vi "HFRR ADV v024 new software.vi"() -> ()   [LabVIEW 2025] (continued)
              n2182 = Fract/Exp String To Number(string=w2595) -> (number=w2598:dbl)  [unwired: 3 in, 1 out]
              n2183 = Add(x=w2598, y=0.0) -> (x+y=w2594:dbl)
            }
            n2184 = for {
              N: w2486 -> [_]
              tunnel: w2493 -> [w2541]
              tunnel: w2492 -> [w2540]
              tunnel: [w2530] -> w2446 mode=indexing
              tunnel: [w2529] -> w2439 mode=indexing
              tunnel: w2483 -> [_]
              tunnel: [w2518] -> w2444 mode=indexing
              tunnel: [w2523] -> w2441 mode=indexing
              tunnel: [w2519] -> w2431 mode=indexing
              tunnel: [w2514] -> w2406 mode=indexing
              tunnel: [w2510] -> w2387 mode=indexing
              tunnel: [w2505] -> w2347 mode=indexing
              (unwired) 1.0 ("x")
              (unwired) TRUE ("line mode (F)")
              n2185 = Read from Text File "Read File"(file (use dialog)=w2541, error in=w2540) -> (text=w2506:string)  [unwired: 2 in, 3 out]
              n2186 = local write "String 12"(w2506) -> ()
              n2187 = String Subset(string=w2506, offset (0)=85, length (rest)=9 ("length (rest)")) -> (substring=w2508:string)
              n2188 = String Subset(string=w2506, offset (0)=35, length (rest)=9 ("length (rest)")) -> (substring=w2531:string)
              n2189 = String Subset(string=w2506, offset (0)=55, length (rest)=9 ("length (rest)")) -> (substring=w2516:string)
              n2190 = String Subset(string=w2506, offset (0)=25, length (rest)=9 ("length (rest)")) -> (substring=w2512:string)
              n2191 = String Subset(string=w2506, offset (0)=45, length (rest)=9 ("length (rest)")) -> (substring=w2521:string)
              n2192 = String Subset(string=w2506, offset (0)=15, length (rest)=9 ("length (rest)")) -> (substring=w2537:string)
              n2193 = String Subset(string=w2506, offset (0)=0, length (rest)=14 ("length (rest)")) -> (substring=w2534:string)
              n2194 = String Subset(string=w2506, offset (0)=65, length (rest)=9 ("length (rest)")) -> (substring=w2524:string)
              n2195 = Fract/Exp String To Number(string=w2508) -> (number=w2505:dbl)  [unwired: 3 in, 1 out]
              n2196 = Fract/Exp String To Number(string=w2531) -> (number=w2529:dbl)  [unwired: 3 in, 1 out]
              n2197 = Fract/Exp String To Number(string=w2516) -> (number=w2514:dbl)  [unwired: 3 in, 1 out]
              n2198 = Fract/Exp String To Number(string=w2512) -> (number=w2510:dbl)  [unwired: 3 in, 1 out]
              n2199 = Fract/Exp String To Number(string=w2521) -> (number=w2519:dbl)  [unwired: 3 in, 1 out]
              n2200 = Fract/Exp String To Number(string=w2537) -> (number=w2518:dbl)  [unwired: 3 in, 1 out]
              n2201 = Fract/Exp String To Number(string=w2534) -> (number=w2530:dbl)  [unwired: 3 in, 1 out]
              n2202 = Fract/Exp String To Number(string=w2524) -> (number=w2527:dbl)  [unwired: 3 in, 1 out]
              n2203 = Add(x=w2527, y=0.0) -> (x+y=w2523:dbl)
            }
            n2204 = Delete From Array(array=w2389, index=0) -> (array with subset deleted=w2362:dbl[])  [unwired: 1 in, 1 out]
            n2205 = Delete From Array(array=w2452, index=0) -> (array with subset deleted=w2425:dbl[])  [unwired: 1 in, 1 out]
            n2206 = Delete From Array(array=w2432, index=0) -> (array with subset deleted=w2420:dbl[])  [unwired: 1 in, 1 out]
            n2207 = Delete From Array(array=w2450, index=0) -> (array with subset deleted=w2451:dbl[])  [unwired: 1 in, 1 out]
            n2208 = call-poly <vilib>:"Mean.vi"("X"=w2362) -> ("mean"=→"КОФ2 4":dbl)  [unwired: 1 out]
            n2209 = call-poly <vilib>:"Mean.vi"("X"=w2425) -> ("mean"=→"КОФ3":dbl)  [unwired: 1 out]
            n2210 = call-poly <vilib>:"Mean.vi"("X"=w2420) -> ("mean"=→"CP3":dbl)  [unwired: 1 out]
            n2211 = Delete From Array(array=w2414, index=0) -> (array with subset deleted=w2341:dbl[])  [unwired: 1 in, 1 out]
            n2212 = Delete From Array(array=w2353, index=0) -> (array with subset deleted=w2340:dbl[])  [unwired: 1 in, 1 out]
            n2213 = Delete From Array(array=w2393, index=0) -> (array with subset deleted=w2364:dbl[])  [unwired: 1 in, 1 out]
            n2214 = Delete From Array(array=w2471, index=0) -> (array with subset deleted=w2426:dbl[])  [unwired: 1 in, 1 out]
            n2215 = Delete From Array(array=w2437, index=0) -> (array with subset deleted=w2422:dbl[])  [unwired: 1 in, 1 out]
            "array w/ subset deleted" <- w2422
            n2216 = Delete From Array(array=w2468, index=0) -> (array with subset deleted=w2469:dbl[])  [unwired: 1 in, 1 out]
            n2217 = call-poly <vilib>:"Mean.vi"("X"=w2364) -> ("mean"=→"КОФ2 2":dbl)  [unwired: 1 out]
            n2218 = call-poly <vilib>:"Mean.vi"("X"=w2426) -> ("mean"=→"КОФ1":dbl)  [unwired: 1 out]
            n2219 = Bundle "Bundle"(w2341, w2340) -> (w2346:cluster{dbl[], dbl[]})  [unwired: 1 in]
            n2220 = Bundle "Bundle"(w2341, w2469) -> (w2333:cluster{dbl[], dbl[]})  [unwired: 1 in]
            n2221 = Delete From Array(array=w2348, index=0) -> (array with subset deleted=w2336:dbl[])  [unwired: 1 in, 1 out]
            n2222 = Delete From Array(array=w2349, index=0) -> (array with subset deleted=w2338:dbl[])  [unwired: 1 in, 1 out]
            n2223 = Delete From Array(array=w2459, index=0) -> (array with subset deleted=w2460:dbl[])  [unwired: 1 in, 1 out]
            n2224 = Delete From Array(array=w2347, index=0) -> (array with subset deleted=w2334:dbl[])  [unwired: 1 in, 1 out]
            n2225 = Delete From Array(array=w2441, index=0) -> (array with subset deleted=w2442:dbl[])  [unwired: 1 in, 1 out]
            n2226 = Delete From Array(array=w2466, index=0) -> (array with subset deleted=w2372:dbl[])  [unwired: 1 in, 1 out]
            n2227 = Delete From Array(array=w2412, index=0) -> (array with subset deleted=w2368:dbl[])  [unwired: 1 in, 1 out]
            n2228 = Delete From Array(array=w2448, index=0) -> (array with subset deleted=w2370:dbl[])  [unwired: 1 in, 1 out]
            n2229 = Delete From Array(array=w2408, index=0) -> (array with subset deleted=w2366:dbl[])  [unwired: 1 in, 1 out]
            n2230 = Delete From Array(array=w2457, index=0) -> (array with subset deleted=w2371:dbl[])  [unwired: 1 in, 1 out]
            n2231 = Delete From Array(array=w2410, index=0) -> (array with subset deleted=w2367:dbl[])  [unwired: 1 in, 1 out]
            n2232 = Delete From Array(array=w2391, index=0) -> (array with subset deleted=w2363:dbl[])  [unwired: 1 in, 1 out]
            n2233 = Delete From Array(array=w2435, index=0) -> (array with subset deleted=w2421:dbl[])  [unwired: 1 in, 1 out]
            n2234 = Delete From Array(array=w2462, index=0) -> (array with subset deleted=w2423:dbl[])  [unwired: 1 in, 1 out]
            n2235 = Delete From Array(array=w2439, index=0) -> (array with subset deleted=w2369:dbl[])  [unwired: 1 in, 1 out]
            n2236 = Delete From Array(array=w2406, index=0) -> (array with subset deleted=w2365:dbl[])  [unwired: 1 in, 1 out]
            n2237 = Delete From Array(array=w2387, index=0) -> (array with subset deleted=w2361:dbl[])  [unwired: 1 in, 1 out]
            n2238 = Delete From Array(array=w2431, index=0) -> (array with subset deleted=w2419:dbl[])  [unwired: 1 in, 1 out]
            n2239 = Delete From Array(array=w2444, index=0) -> (array with subset deleted=w2424:dbl[])  [unwired: 1 in, 1 out]
            n2240 = Delete From Array(array=w2454, index=0) -> (array with subset deleted=w2337:dbl[])  [unwired: 1 in, 1 out]
            n2241 = Delete From Array(array=w2464, index=0) -> (array with subset deleted=w2339:dbl[])  [unwired: 1 in, 1 out]
            n2242 = Delete From Array(array=w2446, index=0) -> (array with subset deleted=w2335:dbl[])  [unwired: 1 in, 1 out]
            n2243 = Bundle "Bundle"(w2341, w2372) -> (w2359:cluster{dbl[], dbl[]})  [unwired: 1 in]
            n2244 = Bundle "Bundle"(w2341, w2426) -> (w2360:cluster{dbl[], dbl[]})  [unwired: 1 in]
            n2245 = Bundle "Bundle"(w2372, w2368) -> (w2374:cluster{dbl[], dbl[]})  [unwired: 1 in]
            n2246 = Bundle "Bundle"(w2337, w2336) -> (w2344:cluster{dbl[], dbl[]})  [unwired: 1 in]
            n2247 = Bundle "Bundle"(w2370, w2366) -> (w2376:cluster{dbl[], dbl[]})  [unwired: 1 in]
            n2248 = Bundle "Bundle"(w2337, w2370) -> (w2480:cluster{dbl[], dbl[]})  [unwired: 1 in]
            n2249 = Bundle "Bundle"(w2337, w2366) -> (w2404:cluster{dbl[], dbl[]})  [unwired: 1 in]
            n2250 = Bundle "Bundle"(w2337, w2425) -> (w2490:cluster{dbl[], dbl[]})  [unwired: 1 in]
            n2251 = Bundle "Bundle"(w2337, w2420) -> (w2428:cluster{dbl[], dbl[]})  [unwired: 1 in]
            n2252 = Bundle "Bundle"(w2337, w2451) -> (w2475:cluster{dbl[], dbl[]})  [unwired: 1 in]
            n2253 = Bundle "Bundle"(w2371, w2367) -> (w2375:cluster{dbl[], dbl[]})  [unwired: 1 in]
            n2254 = Bundle "Bundle"(w2339, w2338) -> (w2345:cluster{dbl[], dbl[]})  [unwired: 1 in]
            n2255 = Bundle "Bundle"(w2339, w2371) -> (w2482:cluster{dbl[], dbl[]})  [unwired: 1 in]
            n2256 = Bundle "Bundle"(w2339, w2367) -> (w2405:cluster{dbl[], dbl[]})  [unwired: 1 in]
            n2257 = Bundle "Bundle"(w2339, w2421) -> (w2429:cluster{dbl[], dbl[]})  [unwired: 1 in]
            n2258 = Bundle "Bundle"(w2339, w2423) -> (w2491:cluster{dbl[], dbl[]})  [unwired: 1 in]
            n2259 = Bundle "Bundle"(w2339, w2460) -> (w2473:cluster{dbl[], dbl[]})  [unwired: 1 in]
            n2260 = Bundle "Bundle"(w2369, w2365) -> (w2377:cluster{dbl[], dbl[]})  [unwired: 1 in]
            n2261 = Bundle "Bundle"(w2335, w2334) -> (w2343:cluster{dbl[], dbl[]})  [unwired: 1 in]
            n2262 = Bundle "Bundle"(w2335, w2369) -> (w2481:cluster{dbl[], dbl[]})  [unwired: 1 in]
            n2263 = Bundle "Bundle"(w2335, w2365) -> (w2403:cluster{dbl[], dbl[]})  [unwired: 1 in]
            n2264 = Bundle "Bundle"(w2335, w2419) -> (w2427:cluster{dbl[], dbl[]})  [unwired: 1 in]
            n2265 = Bundle "Bundle"(w2335, w2424) -> (w2489:cluster{dbl[], dbl[]})  [unwired: 1 in]
            n2266 = Bundle "Bundle"(w2335, w2442) -> (w2474:cluster{dbl[], dbl[]})  [unwired: 1 in]
            n2267 = call-poly <vilib>:"Mean.vi"("X"=w2422) -> ("mean"=→"CP1":dbl)  [unwired: 1 out]
            n2268 = call-poly <vilib>:"Mean.vi"("X"=w2363) -> ("mean"=→"КОФ2 3":dbl)  [unwired: 1 out]
            n2269 = call-poly <vilib>:"Mean.vi"("X"=w2421) -> ("mean"=→"CP2":dbl)  [unwired: 1 out]
            n2270 = call-poly <vilib>:"Mean.vi"("X"=w2423) -> ("mean"=→"КОФ2":dbl)  [unwired: 1 out]
            n2271 = call-poly <vilib>:"Mean.vi"("X"=w2361) -> ("mean"=→"КОФ2 5":dbl)  [unwired: 1 out]
            n2272 = call-poly <vilib>:"Mean.vi"("X"=w2419) -> ("mean"=→"CP4":dbl)  [unwired: 1 out]
            n2273 = call-poly <vilib>:"Mean.vi"("X"=w2424) -> ("mean"=→"КОФ4":dbl)  [unwired: 1 out]
            n2274 = Bundle "Bundle"(w2341, w2368) -> (w2332:cluster{dbl[], dbl[]})  [unwired: 1 in]
            n2275 = Bundle "Bundle"(w2341, w2422) -> (w2355:cluster{dbl[], dbl[]})  [unwired: 1 in]
            n2276 = Build Array "Build Array"(w2332, w2355) -> (w2358:cluster{dbl[], dbl[]}[])
            "XY Graph 17" <- w2358
            n2277 = Build Array "Build Array"(w2346, w2345, w2344, w2343) -> (→"Frequency ( Hz )":cluster{dbl[], dbl[]}[])
            n2278 = Build Array "Build Array"(w2374, w2375, w2376, w2377) -> (→"Air Temp ( °C ) vs Humidity ( % RH )":cluster{dbl[], dbl[]}[])
            n2279 = Build Array "Build Array"(w2359, w2482, w2480, w2481) -> (→"Air Temperature  ( °C )":cluster{dbl[], dbl[]}[])
            n2280 = Build Array "Build Array"(w2332, w2405, w2404, w2403) -> (→"Humidity ( %RH )":cluster{dbl[], dbl[]}[])
            n2281 = Build Array "Build Array"(w2360, w2491, w2490, w2489) -> (→"Coefficient Of Friction":cluster{dbl[], dbl[]}[])
            n2282 = Build Array "Build Array"(w2355, w2429, w2428, w2427) -> (→"Sample Temperature ( °C )":cluster{dbl[], dbl[]}[])
            n2283 = Build Array "Build Array"(w2333, w2473, w2475, w2474) -> (→"XY Graph 13":cluster{dbl[], dbl[]}[])
            n2284 = Bundle "Bundle"(w2341, w2364) -> (w2386:cluster{dbl[], dbl[]})  [unwired: 1 in]
            n2285 = Bundle "Bundle"(w2337, w2362) -> (w2384:cluster{dbl[], dbl[]})  [unwired: 1 in]
            n2286 = Bundle "Bundle"(w2339, w2363) -> (w2385:cluster{dbl[], dbl[]})  [unwired: 1 in]
            n2287 = Bundle "Bundle"(w2335, w2361) -> (w2383:cluster{dbl[], dbl[]})  [unwired: 1 in]
            n2288 = Build Array "Build Array"(w2386, w2385, w2384, w2383) -> (→"Stroke ( mm )":cluster{dbl[], dbl[]}[])
            n2289 = local write "XY Graph 16"(w2358) -> ()
          }
          frame #2 {
          }
          frame #3 {
            n2290 = local write "Numeric 8"(0 ("Numeric 8")) -> ()
            n2291 = local write "Numeric 11"(0 ("Numeric 11")) -> ()
            n2292 = local write "Numeric 12"(0 ("Numeric 12")) -> ()
            n2293 = local write "Numeric 13"(0 ("Numeric 13")) -> ()
            n2294 = property on="OPEN" class="Bool (strict)"("Visible"=TRUE) -> ()  [unwired: 2 in, 2 out]
            n2295 = local read "String Control 2"() -> (w2658:string)
            n2296 = local read "String Control 4"() -> (w2657:string)
            n2297 = local read "String Control 6"() -> (w2656:string)
            n2298 = local read "String Control 8"() -> (w2655:string)
            n2299 = Match Pattern(string=w2658, regular expression="Samples / cycle :- ") -> (after substring=w2672:string)  [unwired: 1 in, 3 out]
            n2300 = Match Pattern(string=w2658, regular expression="Frequency :- ") -> (after substring=w2691:string)  [unwired: 1 in, 3 out]
            n2301 = Match Pattern(string=w2657, regular expression="Samples / cycle :- ") -> (after substring=w2668:string)  [unwired: 1 in, 3 out]
            n2302 = Match Pattern(string=w2657, regular expression="Frequency :- ") -> (after substring=w2686:string)  [unwired: 1 in, 3 out]
            n2303 = Match Pattern(string=w2656, regular expression="Samples / cycle :- ") -> (after substring=w2664:string)  [unwired: 1 in, 3 out]
            n2304 = Match Pattern(string=w2656, regular expression="Frequency :- ") -> (after substring=w2681:string)  [unwired: 1 in, 3 out]
            n2305 = Match Pattern(string=w2655, regular expression="Samples / cycle :- ") -> (after substring=w2660:string)  [unwired: 1 in, 3 out]
            n2306 = Match Pattern(string=w2655, regular expression="Frequency :- ") -> (after substring=w2676:string)  [unwired: 1 in, 3 out]
            n2307 = String Subset(string=w2672, length (rest)=6 ("length (rest)")) -> (substring=w2674:string)  [unwired: 1 in]
            n2308 = String Subset(string=w2691, length (rest)=9 ("length (rest)")) -> (substring=w2693:string)  [unwired: 1 in]
            n2309 = String Subset(string=w2668, length (rest)=6 ("length (rest)")) -> (substring=w2670:string)  [unwired: 1 in]
            n2310 = String Subset(string=w2686, length (rest)=9 ("length (rest)")) -> (substring=w2688:string)  [unwired: 1 in]
            n2311 = String Subset(string=w2664, length (rest)=6 ("length (rest)")) -> (substring=w2666:string)  [unwired: 1 in]
            n2312 = String Subset(string=w2681, length (rest)=9 ("length (rest)")) -> (substring=w2683:string)  [unwired: 1 in]
            n2313 = String Subset(string=w2660, length (rest)=6 ("length (rest)")) -> (substring=w2662:string)  [unwired: 1 in]
            n2314 = String Subset(string=w2676, length (rest)=9 ("length (rest)")) -> (substring=w2678:string)  [unwired: 1 in]
            n2315 = Fract/Exp String To Number(string=w2674) -> (number=w2654:dbl)  [unwired: 3 in, 1 out]
            n2316 = Fract/Exp String To Number(string=w2693) -> (number=w2694:dbl)  [unwired: 3 in, 1 out]
            n2317 = Fract/Exp String To Number(string=w2670) -> (number=w2653:dbl)  [unwired: 3 in, 1 out]
            n2318 = Fract/Exp String To Number(string=w2688) -> (number=w2689:dbl)  [unwired: 3 in, 1 out]
            n2319 = Fract/Exp String To Number(string=w2666) -> (number=w2652:dbl)  [unwired: 3 in, 1 out]
            n2320 = Fract/Exp String To Number(string=w2683) -> (number=w2684:dbl)  [unwired: 3 in, 1 out]
            n2321 = Fract/Exp String To Number(string=w2662) -> (number=w2651:dbl)  [unwired: 3 in, 1 out]
            n2322 = Fract/Exp String To Number(string=w2678) -> (number=w2679:dbl)  [unwired: 3 in, 1 out]
            n2323 = local write "sample1"(w2654) -> ()
            n2324 = local write "freq1"(w2694) -> ()
            n2325 = local write "sample2"(w2653) -> ()
            n2326 = local write "freq2"(w2689) -> ()
            n2327 = local write "sample3"(w2652) -> ()
            n2328 = local write "freq3"(w2684) -> ()
            n2329 = local write "sample4"(w2651) -> ()
            n2330 = local write "freq 4"(w2679) -> ()
          }
        }
      }
    }
    n2331 = case shown="True" w2143 {
      selector: w2143 -> [_ w2271]
      frame False {
      }
      frame True {
        n2332 = Not(x=w2271) -> (.not. x?=w2267:bool)
        n2333 = local write "service 3"(w2267) -> ()
        n2334 = local write "OPEN 6"(w2267) -> ()
        n2335 = call <vilib>:"System Exec.vi"("wait until completion? (T)"=TRUE, "command line"="C:\\LAB-IQ\\Scar View.exe") -> ("error out"=→"error out 5":errorcluster)  [unwired: 6 in, 3 out]
      }
    }
    n2336 = case shown="\"Acquire\", Default" w2154 {
      frame "Acquire", Default {
        w3160 = 0.2 ("y")
        w3165 = 1.0 ("y")
        w3166 = 0.8 ("y")
        # "Elapsed time\ncof\nstroke\nAir temp\nTemp\nHumidity"
        n2337 = disable-structure shown="Disabled" {
          frame Disabled {
            n2338 = local read "Flag"() -> (w3183:dbl)
            n2339 = local read "RUN"() -> (w3180:bool)
            n2340 = Not(x=w3180) -> (.not. x?=w3179:bool)
            n2341 = Equal?(x=w3183, y=10.0) -> (x = y?=w3181:bool)
            n2342 = And(x=w3181, y=w3179) -> (x .and. y?=w3178:bool)
            n2343 = case shown="True" w3178 {
              frame False {
              }
              frame True {
                w3184 = FALSE ("Heater Button")
                n2344 = local write "Humidity"(w3184) -> ()
                n2345 = local write "Heater Button"(w3184) -> ()
              }
            }
          }
          frame Enabled {
          }
        }
        n2346 = disable-structure shown="Disabled" {
          frame Disabled {
            n2347 = case shown="True" {
              selector: _ -> [_ _]
              frame False {
              }
              frame True {
                w3275 = TRUE ("Heater")
                n2348 = local write "Humidity"(w3275) -> ()
                n2349 = local write "Heater Button"(w3275) -> ()
                n2350 = local read "TEST STANDARD"() -> (w3278:T3)
                n2351 = local read "TEST STANDARD"() -> (w3273:T3)
                n2352 = Equal?(x=w3278, y=enum16{"ASTM D6079", "ISO 12156", "Custom"}."ISO 12156" ("Test Standard")) -> (x = y?=w3276:bool)
                n2353 = Equal?(x=w3273, y=enum16{"ASTM D6079", "ISO 12156", "Custom"}."ASTM D6079" ("Test Standard")) -> (x = y?=w3272:bool)
                n2354 = case shown="True" w3276 {
                  frame False {
                  }
                  frame True {
                    n2355 = local write "Heater"(TRUE ("Heater")) -> ()
                    n2356 = local write "airtempflg"(FALSE ("airtempflg")) -> ()
                  }
                }
                n2357 = case shown="True" w3272 {
                  frame False {
                  }
                  frame True {
                    n2358 = local write "Heater"(FALSE ("Heater")) -> ()
                    n2359 = local write "airtempflg"(TRUE ("airtempflg")) -> ()
                  }
                }
              }
            }
          }
          frame Enabled {
          }
        }
        n2360 = stacked-sequence {
          frame #0 {
            n2361 = case shown="True" "RST FF" {
              frame False {
              }
              frame True {
                w3341 = 0.0 ("X Scale.Range:Maximum")
                n2362 = property on="Frictional Force ( N )" class="WFChart (strict)"("XScale.Maximum"=600.0 ("X Scale.Range:Maximum"), "XScale.Minimum"=w3341, "YScale.Maximum"=10.0 ("Y Scale.Range:Maximum"), "YScale.Minimum"=w3341) -> ()  [unwired: 2 in, 2 out]
              }
            }
          }
          frame #1 {
            n2363 = case shown="True" "RST TEMP" {
              frame False {
              }
              frame True {
                n2364 = property on="Temperature ( Deg C )" class="WFChart (strict)"("XScale.Minimum"=0.0 ("X Scale.Range:Minimum"), "XScale.Maximum"=600.0 ("X Scale.Range:Maximum"), "YScale.Minimum"=0.0 ("Y Scale.Range:Minimum"), "YScale.Maximum"=100.0 ("Y Scale.Range:Maximum")) -> ()  [unwired: 2 in, 2 out]
              }
            }
          }
          frame #2 {
            n2365 = case shown="True" "RSTCOF" {
              frame False {
              }
              frame True {
                n2366 = property on="Coefficient of Friction" class="WFChart (strict)"("XScale.Minimum"=0.0 ("X Scale.Range:Minimum"), "XScale.Maximum"=600.0 ("X Scale.Range:Maximum"), "YScale.Maximum"=1.0 ("X Scale.Range:Minimum"), "YScale.Minimum"=0.0 ("X Scale.Range:Minimum")) -> ()  [unwired: 2 in, 2 out]
              }
            }
          }
          frame #3 {
            n2367 = case shown="True" "RSTCOF 2" {
              frame False {
              }
              frame True {
                (unwired) 100.0 ("Y Scale.Range:Maximum")
                (unwired) 0.0 ("Y Scale.Range:Minimum")
                (unwired) 600.0 ("X Scale.Range:Maximum")
                (unwired) 0.0 ("X Scale.Range:Minimum")
              }
            }
          }
          frame #4 {
            n2368 = case shown="True" "RSTCOF 3" {
              frame False {
              }
              frame True {
                n2369 = property on="Electrical Contact Resistance ( % )" class="WFChart (strict)"("XScale.Minimum"=0.0 ("X Scale.Range:Minimum"), "XScale.Maximum"=600.0 ("X Scale.Range:Maximum"), "YScale.Minimum"=0.0 ("Y Scale.Range:Minimum"), "YScale.Maximum"=100.0 ("Y Scale.Range:Maximum")) -> ()  [unwired: 2 in, 2 out]
              }
            }
          }
        }
        n2370 = disable-structure shown="Disabled" {
          frame Disabled {
            n2371 = case shown="True" {
              selector: _ -> [_ _]
              frame False {
              }
              frame True {
                n2372 = local read "zflag 2"() -> (w3242:dbl)
                n2373 = local read "yflag"() -> (w3244:dbl)
                n2374 = Equal?(x=w3244, y=2.0 ("tflag")) -> (x = y?=w3246:bool)
                n2375 = Equal?(x=w3242, y=3.0 ("tflag")) -> (x = y?=w3245:bool)
                n2376 = And(x=w3246, y=w3245) -> (x .and. y?=w3240:bool)
                n2377 = case shown="True" w3240 {
                  frame False {
                  }
                  frame True {
                    w3271 = 0.0 ("zflag")
                    n2378 = local write "zflag"(w3271) -> ()
                    n2379 = local write "zflag 2"(w3271) -> ()
                    n2380 = Delete(path (use dialog)=path "C:/LAB-IQ-NXT/WO 2449 TT.sig" ("file path (dialog if empty)")) -> (deleted path=w3270:path)  [unwired: 4 in, 2 out]
                    n2381 = Delete(path (use dialog)=path "C:/LAB-IQ-NXT/WO 2449 TRH.sig" ("file path (dialog if empty)")) -> (deleted path=w3265:path)  [unwired: 4 in, 2 out]
                    n2382 = local read "SEN.RUN HRS"() -> (w3257:dbl)
                    n2383 = local read "SENSOR TIME"() -> (w3255:dbl)
                    n2384 = call <vilib>:"compatOverwrite.vi"("overwrite (F)"=TRUE) -> ("overwrite?"=w3247:T30)
                    n2385 = call <vilib>:"compatOverwrite.vi"("overwrite (F)"=TRUE) -> ("overwrite?"=w3251:T30)
                    n2386 = local read "Total No. of Tests"() -> (w3258:dbl)
                    n2387 = Add(x=w3255, y=w3257) -> (x+y=w3256:dbl)
                    "SEN.RUN HRS" <- w3256
                    n2388 = Open/Create/Replace File(file path (use dialog)=w3270, operation (0:open)=w3247) -> (refnum out=w3248:refnum<file>, error out=w3249:errorcluster)  [unwired: 4 in, 1 out]
                    n2389 = Open/Create/Replace File(file path (use dialog)=w3265, operation (0:open)=w3251) -> (refnum out=w3252:refnum<file>, error out=w3253:errorcluster)  [unwired: 4 in, 1 out]
                    n2390 = Deny Access(4:w3249, 6:T28."deny none" ("deny mode (2)"), 7:w3248) -> (3:w3269:refnum<file>)  [unwired: 1 out]
                    n2391 = Deny Access(4:w3253, 6:T28."deny none" ("deny mode (2)"), 7:w3252) -> (3:w3261:refnum<file>)  [unwired: 1 out]
                    n2392 = Number To Decimal String(number=w3258) -> (decimal integer string=w3266:string)  [unwired: 1 in]
                    n2393 = Number To Decimal String(number=w3256) -> (decimal integer string=w3262:string)  [unwired: 1 in]
                    n2394 = Write to Binary File(file (use dialog)=w3269, data=w3266, 5:FALSE ("prepend array or string size? (T)")) -> ()  [unwired: 3 in, 3 out]
                    n2395 = Write to Binary File(file (use dialog)=w3261, data=w3262, 5:FALSE ("prepend array or string size? (T)")) -> ()  [unwired: 3 in, 3 out]
                  }
                }
              }
            }
          }
          frame Enabled {
          }
        }
        n2396 = local read "RUN"() -> (w3169:bool)
        n2397 = local read "run replace"() -> (w3173:bool)
        n2398 = local read "run replace"() -> (w3172:bool)
        n2399 = case shown="True" w3169 {
          frame False {
            n2400 = local write "run replace"(FALSE ("run replace")) -> ()
          }
          frame True {
            "run replace" <- TRUE ("run replace")
          }
        }
        n2401 = local read "RUN"() -> (w3177:bool)
        n2402 = local read "Set Temp"() -> (w3139:dbl)
        n2403 = local read "SetTemp"() -> (w3141:dbl)
        n2404 = case shown="False" w3177 {
          tunnel: [FALSE ("TEST RUNNING") TRUE ("TEST RUNNING")] -> w3176
          frame False {
            w3360 = 0.0 ("Flag")
            n2405 = local write "Elapsed time"(0.0 ("elapsedtime")) -> ()
            n2406 = local write "Time Remaining"(w3360) -> ()
            n2407 = local write "Flag"(w3360) -> ()
            n2408 = local write "Remaining Time"(w3360) -> ()
          }
          frame True {
            n2409 = local write "Flag"(10.0 ("Flag")) -> ()
          }
        }
        n2410 = case shown="False" w3173 {
          frame False {
            n2411 = local read "zflag"() -> (→"zflag 2":dbl)
            n2412 = local write "yflag"(2.0 ("tflag")) -> ()
            n2413 = local write "FLAG 4"(0.0 ("FLAG")) -> ()
          }
          frame True {
            n2414 = local write "yflag"(1.0 ("tflag")) -> ()
            n2415 = local write "zflag"(3.0 ("zflag")) -> ()
          }
        }
        n2416 = local read "acq 2"() -> (w3171:bool)
        n2417 = local read "AIR TEMP"() -> (w3134:dbl)
        n2418 = local read "Amb temp"() -> (w3138:dbl)
        n2419 = case shown="True" "Save & Continue" {
          frame False {
          }
          frame True {
            "acq 2" <- TRUE ("acq 2")
          }
        }
        n2420 = local read "Set Rh"() -> (w3140:dbl)
        n2421 = Add(x=w3141, y=w3166) -> (x+y=w3167:dbl)
        n2422 = Subtract(x=w3141, y=w3166) -> (x-y=w3168:dbl)
        n2423 = Add(x=w3139, y=w3160) -> (x+y=w3161:dbl)
        n2424 = Subtract(x=w3139, y=w3160) -> (x-y=w3162:dbl)
        n2425 = And(x=w3171, y=w3172) -> (x .and. y?=w3170:bool)
        n2426 = Greater Or Equal?(x=w3134, y=15.0) -> (x >= y?=w3135:bool)
        "powstat" <- w3135
        n2427 = local read "Humidity ( %RH )"() -> (w3137:dbl)
        n2428 = case shown="True" "Save & Continue" {
          frame False {
          }
          frame True {
            n2429 = while {
              tunnel: "0123456789abcdefghijklmnopqrstuvwxyzABCDEFGHIJKLMNOPQRSTUVWXYZ" ("string 2") -> [w3331]
              shift-right: [w3329] -> w3324
              shift-left: "" -> [w3328]
              i -> [w3338]
              stop <- w3337 stop-if-true
              n2430 = Random Number (0-1)() -> (number: 0 to 1=w3332:dbl)
              n2431 = Multiply(x=w3332, y=62.0) -> (x*y=w3334:dbl)
              n2432 = Decrement(x="Length") -> (x-1=w3327:i16)
              n2433 = To Word Integer(number=w3334) -> (16bit integer=w3335:i16)
              n2434 = String Subset(string=w3331, offset (0)=w3335, length (rest)=1 ("length (rest)")) -> (substring=w3330:string)
              n2435 = Greater Or Equal?(x=w3338, y=w3327) -> (x >= y?=w3337:bool)
              n2436 = Concatenate Strings(w3330, w3328) -> (w3329:string)
            }
            n2437 = local write "UUID"(w3324) -> ()
          }
        }
        n2438 = In Range and Coerce(upper limit=w3167, x=w3138, lower limit=w3168) -> (In Range?=w3157:bool)  [unwired: 1 out]
        n2439 = Add(x=w3140, y=w3165) -> (x+y=w3164:dbl)
        n2440 = Subtract(x=w3140, y=w3165) -> (x-y=w3163:dbl)
        n2441 = local read "TEMP"() -> (w3136:dbl)
        n2442 = case shown="True" "Save & Continue" {
          frame False {
          }
          frame True {
            n2443 = local read "Operator ID"() -> (w3655:string)
            n2444 = local read "FILE"() -> (w3661:string)
            n2445 = String Length(string=w3661) -> (length=w3659:i32)
            n2446 = String Length(string=w3655) -> (length=w3656:i32)
            n2447 = Greater?(x=w3659, y=0) -> (0:w3658:bool)
            n2448 = Greater?(x=w3656, y=0) -> (0:w3654:bool)
            n2449 = And(x=w3658, y=w3654) -> (x .and. y?=w3653:bool)
            n2450 = case shown="True" w3653 {
              frame False {
                n2451 = stacked-sequence {
                  frame #0 {
                    n2452 = One Button Dialog(message="Please Enter a File Name and Operator ID to save data !", button name ("OK")="Ok") -> ()  [unwired: 1 out]
                  }
                  frame #1 {
                    n2453 = local write "Save & Continue"(FALSE ("OK Button")) -> ()
                  }
                }
                n2454 = local write "Save & Continue"(FALSE ("OK Button")) -> ()
              }
              frame True {
                n2455 = stacked-sequence {
                  frame #0 {
                    n2456 = local read "FILE"() -> (w3667:string)
                    n2457 = call "file check.vi"("file name in"=w3667) -> ("file name out"=w3666:string)  [unwired: 9 in, 1 out]
                    n2458 = call <vilib>:"Application Directory.vi"() -> ("Application Directory"=w3677:path)
                    n2459 = Build Path(base path=w3677, name or relative path="data") -> (appended path=w3676:path)
                    n2460 = call <vilib>:"Trim Whitespace.vi"("string"=w3666) -> ("trimmed string"=w3674:string)  [unwired: 1 in]
                    n2461 = call <vilib>:"Trim Whitespace.vi"("string"=w3666) -> ("trimmed string"=w3675:string)  [unwired: 1 in]
                    n2462 = List Folder(path=w3676) -> (folder names=w3672:string[])  [unwired: 3 in, 3 out]
                    n2463 = Match Pattern(string=w3674, regular expression="_(") -> (before substring=w3671:string)  [unwired: 1 in, 3 out]
                    n2464 = for {
                      tunnel: w3672 -> [w3686] mode=indexing
                      tunnel: w3671 -> [w3684]
                      shift-right: [w3682] -> w3669
                      shift-left: bool[] [] -> [w3683]
                      n2465 = Match Pattern(string=w3686, regular expression="_(") -> (before substring=w3685:string)  [unwired: 1 in, 3 out]
                      n2466 = Equal?(x=w3685, y=w3684) -> (x = y?=w3681:bool)
                      n2467 = case shown="True" w3681 {
                        tunnel: w3681 -> [_ w3689]
                        tunnel: w3683 -> [w3688 w3691]
                        tunnel: [w3688 w3690] -> w3682
                        frame False {
                        }
                        frame True {
                          n2468 = Insert Into Array(array=w3691, new element=w3689) -> (w3690:bool[])  [unwired: 1 in]
                        }
                      }
                    }
                    n2469 = Equal?(x=w3672, y=w3671) -> (x = y?=w3680:bool[])
                    n2470 = Or Array Elements(Boolean array=w3680) -> (logical OR=w3679:bool)
                    n2471 = Array Size(array=w3669) -> (size(s)=w3668:i32)
                    n2472 = case shown="True" w3679 {
                      tunnel: w3675 -> [_ w3699]
                      tunnel: w3668 -> [_ w3692]
                      frame False {
                      }
                      frame True {
                        n2473 = Number To Decimal String(number=w3692) -> (decimal integer string=w3695:string)  [unwired: 1 in]
                        n2474 = Search/Split String(string=w3699, search string/char (-)="_(" ("regular expression")) -> (substring before match=w3697:string)  [unwired: 1 in, 2 out]
                        n2475 = Concatenate Strings(w3697, "_(" ("regular expression"), w3695, ")" ("regular expression")) -> (w3693:string)
                        n2476 = local write "FILE"(w3693) -> ()
                      }
                    }
                  }
                  frame #1 {
                    w3701 = 0.0
                    w3714 = cluster{"y":dbl, dbl, "y":dbl}[] [] ("History Data")
                    w3715 = FALSE ("Heater Button")
                    (unwired) ")!" ("string")
                    (unwired) ")" ("string")
                    w3713 = dbl[] [] ("History Data")
                    w3719 = "\r"
                    # "C:\\WinDucom\\Data\\"
                    # "C:\\LAB-IQ-NXT\\data"
                    n2477 = local write "Humidity ( %RH )"(w3701) -> ()
                    n2478 = local write "Frequency ( Hz )"(w3701) -> ()
                    n2479 = local write "Stroke 3"(w3701) -> ()
                    n2480 = local write "speedop"(0.0 ("PIDclk 2")) -> ()
                    n2481 = local write "Set Temp 2"(65.0 ("Set Temp 2")) -> ()
                    n2482 = local write "AIR TEMP"(w3701) -> ()
                    n2483 = local write "clk"(0.0 ("clk")) -> ()
                    n2484 = local write "Stroke 4"(w3701) -> ()
                    n2485 = local write "COF 2"(w3701) -> ()
                    n2486 = local write "TEMP"(w3701) -> ()
                    n2487 = local write "ecr 3"(w3701) -> ()
                    n2488 = local write "FF 3"(w3701) -> ()
                    n2489 = local write "FF 2"(w3701) -> ()
                    n2490 = property on="Humidity ( %RH )" class="WFChart (strict)"("History Data"=w3713) -> ()  [unwired: 2 in, 2 out]
                    n2491 = property on="Coefficient of Friction" class="WFChart (strict)"("History Data"=w3713) -> ()  [unwired: 2 in, 2 out]
                    n2492 = property on="Coefficient of Friction" class="WFChart (strict)"("History Data"=w3713) -> ()  [unwired: 2 in, 2 out]
                    n2493 = property on="Frictional Force ( N )" class="WFChart (strict)"("History Data"=w3713) -> ()  [unwired: 2 in, 2 out]
                    n2494 = property on="Electrical Contact Resistance ( % )" class="WFChart (strict)"("History Data"=w3713) -> ()  [unwired: 2 in, 2 out]
                    n2495 = property on="Electrical Contact Resistance ( % )" class="WFChart (strict)"("History Data"=w3713) -> ()  [unwired: 2 in, 2 out]
                    n2496 = property on="Temperature ( Deg C )" class="WFChart (strict)"("History Data"=w3713) -> ()  [unwired: 2 in, 2 out]
                    n2497 = property on="Frictional Force ( N )" class="WFChart (strict)"("History Data"=w3713) -> ()  [unwired: 2 in, 2 out]
                    n2498 = property on="Coefficient of Friction" class="WFChart (strict)"("History Data"=w3713) -> ()  [unwired: 2 in, 2 out]
                    n2499 = property on="Frictional Force ( N )" class="WFChart (strict)"("History Data"=w3713) -> ()  [unwired: 2 in, 2 out]
                    n2500 = property on="Electrical Contact Resistance ( % )" class="WFChart (strict)"("History Data"=w3713) -> ()  [unwired: 2 in, 2 out]
                    n2501 = property on="Temperature ( Deg C )" class="WFChart (strict)"("History Data"=w3713) -> ()  [unwired: 2 in, 2 out]
                    n2502 = property on="Humidity ( %RH )" class="WFChart (strict)"("History Data"=w3713) -> ()  [unwired: 2 in, 2 out]
                    n2503 = property on="Stroke ( mm )" class="WFChart (strict)"("History Data"=w3714) -> ()  [unwired: 2 in, 2 out]
                    n2504 = property on="Stroke ( mm )" class="WFChart (strict)"("History Data"=w3714) -> ()  [unwired: 2 in, 2 out]
                    n2505 = local write "Humidity"(w3715) -> ()
                    n2506 = local write "Heater Button"(w3715) -> ()
                    n2507 = local read "FILE"() -> (w3709:string)
                    n2508 = disable-structure shown="Enabled" {
                      disable-tunnel: [w3754 _] -> w3700
                      frame Enabled {
                        n2509 = local read "NORMAL LOAD"() -> (w3754:dbl)
                      }
                      frame Disabled {
                      }
                    }
                    n2510 = call "file check.vi"("file name in"=w3709) -> ("error out"=w3712:errorcluster, "file name out"=w3706:string)  [unwired: 9 in]
                    n2511 = call "FILE PATH CREATION.vi"("error in"=w3712, "FILE NAME :"=w3706) -> ("FILE OUT"=w3705:path)  [unwired: 8 in, 1 out]
                    n2512 = Concatenate Strings(w3706, ".dgf" ("Substring")) -> (w3711:string)
                    n2513 = Concatenate Strings(w3706, ".duf" ("Substring")) -> (w3707:string)
                    n2514 = Multiply(x=w3700, y=1.0) -> (x*y=w3733:dbl)
                    n2515 = Build Path(base path=w3705, name or relative path=w3711) -> (appended path=w3704:path)
                    n2516 = Build Path(base path=w3705, name or relative path=w3707) -> (appended path=w3703:path)
                    n2517 = Number To Fractional String(number=w3733, width (-)=i16 5, precision (6)=i16 2) -> (F-format string=w3741:string)  [unwired: 1 in]
                    n2518 = local read "Fuel Discription :"() -> (w3729:string)
                    n2519 = local read "Batch Ref Num :"() -> (w3717:string)
                    n2520 = Get Date/Time String(date format (0)=enum16{"short", "long", "abbreviated"}."short") -> (date string=w3752:string, time string=w3749:string)  [unwired: 2 in]
                    n2521 = local read "Remarks :"() -> (w3728:string)
                    n2522 = Concatenate Strings("Load :- " ("Substring"), w3741, " grams ," ("Substring")) -> (w3740:string)
                    n2523 = local read "String 41"() -> (w3720:string)
                    n2524 = Concatenate Strings(w3729) -> (w3730:string)
                    n2525 = Concatenate Strings(w3717) -> (w3716:string)
                    n2526 = Concatenate Strings("tested by") -> (w3724:string)
                    n2527 = Concatenate Strings("(" ("Substring"), w3752, ")" ("Substring"), w3749) -> (w3722:string)
                    "concatenated string" <- w3722
                    n2528 = Concatenate Strings(w3728, "," ("string")) -> (w3727:string)
                    n2529 = Concatenate Strings("  TIME;      COF;       STROKE;     AIR TEMP;  TEMP;  HUMIDITY;  ECR; PID-OUT; FREQUENCY" ("Substring"), "\r") -> (w3736:string)
                    n2530 = Concatenate Strings(w3720, w3719, "Fuel Discription :-" ("Substring"), w3730, w3719, w3740, w3719, "Batch Ref Num :-" ("Substring"), w3716, w3719, " Remarks :- " ("Substring"), w3727, w3719, " Date :- " ("Substring"), w3722, w3719, "Tested By :-" ("Substring"), w3724) -> (w3734:string)
                    "REMARKS" <- w3734
                    n2531 = call <vilib>:"Write Characters To File.vi"("append to file? (new file:F)"=FALSE, "character string"=w3736, "file path (dialog if empty)"=w3704) -> ()  [unwired: 2 in, 1 out]
                    n2532 = call <vilib>:"Write Characters To File.vi"("append to file? (new file:F)"=FALSE, "character string"=w3734, "file path (dialog if empty)"=w3703) -> ()  [unwired: 2 in, 1 out]
                  }
                  frame #2 {
                    n2533 = local write "Cycles elapsed"(0 ("Cycles elapsed")) -> ()
                    n2534 = local write "cyclecount"(0 ("cyclecount")) -> ()
                    n2535 = local write "Save & Continue"(FALSE ("OK")) -> ()
                    n2536 = local write "autostrtflg"(TRUE ("autostrtflg")) -> ()
                    n2537 = local write "Save"(FALSE ("Save")) -> ()
                    n2538 = Get Date/Time In Seconds() -> (seconds since 1Jan1904=w3759:timestamp)
                    n2539 = To Double Precision Float(number=w3759) -> (double precision float=w3758:dbl)
                    n2540 = local write "acq timer"(w3758) -> ()
                    n2541 = One Button Dialog(message="Please ensure sample is mounted properly and machine is ready in all aspects for testing !", button name ("OK")="Ok") -> ()  [unwired: 1 out]
                  }
                  frame #3 {
                    n2542 = stacked-sequence {
                      frame #0 {
                        n2543 = local write "Main Dashboard Buttons"(T1."Dashboard" ("Main Dashboard Buttons")) -> ()
                        n2544 = local write "Main Tab"(T2."Acquire" ("Main Tab")) -> ()
                      }
                      frame #1 {
                        n2545 = local write "EVENT LOG"("" ("EVENT LOG")) -> ()
                      }
                      frame #2 {
                        n2546 = Wait (ms)(milliseconds to wait=u32 50) -> ()  [unwired: 1 out]
                      }
                      frame #3 {
                        n2547 = disable-structure shown="Disabled" {
                          frame Disabled {
                            n2548 = local read "EVENT LOG"() -> (w3771:string)
                            n2549 = call "Event Log.vi"("Content"="Test Details", "EVENT LOG"=w3771) -> ("EVENT LOG"=w3770:string)  [unwired: 8 in, 1 out]
                            n2550 = local write "EVENT LOG"(w3770) -> ()
                          }
                          frame Enabled {
                          }
                        }
                      }
                      frame #4 {
                        n2551 = Wait (ms)(milliseconds to wait=u32 50) -> ()  [unwired: 1 out]
                      }
                      frame #5 {
                        n2552 = local read "FILE"() -> (w3773:string)
                        n2553 = Concatenate Strings("File Name :" ("Content"), w3773) -> (w3774:string)
                        n2554 = local read "EVENT LOG"() -> (w3777:string)
                        n2555 = call "Event Log.vi"("Content"=w3774, "EVENT LOG"=w3777) -> ("EVENT LOG"=w3776:string)  [unwired: 8 in, 1 out]
                        n2556 = local write "EVENT LOG"(w3776) -> ()
                      }
                      frame #6 {
                        n2557 = Wait (ms)(milliseconds to wait=u32 50) -> ()  [unwired: 1 out]
                      }
                      frame #7 {
                        n2558 = local read "Batch Ref Num :"() -> (w3779:string)
                        n2559 = Concatenate Strings("Batch Ref No :" ("Content"), w3779) -> (w3780:string)
                        n2560 = local read "EVENT LOG"() -> (w3783:string)
                        n2561 = call "Event Log.vi"("Content"=w3780, "EVENT LOG"=w3783) -> ("EVENT LOG"=w3782:string)  [unwired: 8 in, 1 out]
                        n2562 = local write "EVENT LOG"(w3782) -> ()
                      }
                      frame #8 {
                        n2563 = Wait (ms)(milliseconds to wait=u32 50) -> ()  [unwired: 1 out]
                      }
                      frame #9 {
                        n2564 = local read "tested by"() -> (w3785:string)
                        n2565 = Concatenate Strings("Tested By :" ("Content"), w3785) -> (w3786:string)
                        n2566 = local read "EVENT LOG"() -> (w3789:string)
                        n2567 = call "Event Log.vi"("Content"=w3786, "EVENT LOG"=w3789) -> ("EVENT LOG"=w3788:string)  [unwired: 8 in, 1 out]
                        n2568 = local write "EVENT LOG"(w3788) -> ()
                      }
                      frame #10 {
                        n2569 = Wait (ms)(milliseconds to wait=u32 50) -> ()  [unwired: 1 out]
                      }
                      frame #11 {
                        n2570 = local read "TEST STANDARD"() -> (w3792:T3)
                        n2571 = case shown="\"ASTM D6079\", Default" w3792 {
                          tunnel: ["ASTM D6079" "ISO 12156" "CEC F-096-A-06" "Custom"] -> w3791
                          frame "ASTM D6079", Default {
                          }
                          frame "ISO 12156" {
                          }
                          frame "CEC F-096-A-06" {
                          }
                          frame "Custom" {
                          }
                        }
                        n2572 = Concatenate Strings("Test Standard :" ("Content"), w3791) -> (w3793:string)
                        n2573 = local read "EVENT LOG"() -> (w3796:string)
                        n2574 = call "Event Log.vi"("Content"=w3793, "EVENT LOG"=w3796) -> ("EVENT LOG"=w3795:string)  [unwired: 8 in, 1 out]
                        n2575 = local write "EVENT LOG"(w3795) -> ()
                      }
                      frame #12 {
                        n2576 = Wait (ms)(milliseconds to wait=u32 50) -> ()  [unwired: 1 out]
                      }
                      frame #13 {
                        n2577 = local read "Fuel Discription :"() -> (w3802:string)
                        n2578 = Concatenate Strings("Fuel Description :" ("Content"), w3802) -> (w3803:string)
                        n2579 = local read "EVENT LOG"() -> (w3806:string)
                        n2580 = call "Event Log.vi"("Content"=w3803, "EVENT LOG"=w3806) -> ("EVENT LOG"=w3805:string)  [unwired: 8 in, 1 out]
                        n2581 = local write "EVENT LOG"(w3805) -> ()
                      }
                      frame #14 {
                        n2582 = Wait (ms)(milliseconds to wait=u32 50) -> ()  [unwired: 1 out]
                      }
                      frame #15 {
                        n2583 = local read "Remarks :"() -> (w3808:string)
                        n2584 = Concatenate Strings("Remarks :" ("Content"), w3808) -> (w3809:string)
                        n2585 = local read "EVENT LOG"() -> (w3812:string)
                        n2586 = call "Event Log.vi"("Content"=w3809, "EVENT LOG"=w3812) -> ("EVENT LOG"=w3811:string)  [unwired: 8 in, 1 out]
                        n2587 = local write "EVENT LOG"(w3811) -> ()
                      }
                      frame #16 {
                        n2588 = Wait (ms)(milliseconds to wait=u32 50) -> ()  [unwired: 1 out]
                      }
                      frame #17 {
                        n2589 = local read "Operator ID"() -> (w3814:string)
                        n2590 = Concatenate Strings("Operator ID :" ("Content"), w3814) -> (w3816:string)
                        n2591 = local read "EVENT LOG"() -> (w3818:string)
                        n2592 = call "Event Log.vi"("Content"=w3816, "EVENT LOG"=w3818) -> ("EVENT LOG"=w3817:string)  [unwired: 8 in, 1 out]
                        n2593 = local write "EVENT LOG"(w3817) -> ()
                      }
                      frame #18 {
                        n2594 = Wait (ms)(milliseconds to wait=u32 50) -> ()  [unwired: 1 out]
                      }
                      frame #19 {
                        n2595 = disable-structure shown="Disabled" {
                          frame Disabled {
                            n2596 = local read "EVENT LOG"() -> (w3822:string)
                            n2597 = call "Event Log.vi"("Content"="Test Parameter", "EVENT LOG"=w3822) -> ("EVENT LOG"=w3821:string)  [unwired: 8 in, 1 out]
                            n2598 = local write "EVENT LOG"(w3821) -> ()
                          }
                          frame Enabled {
                          }
                        }
                      }
                      frame #20 {
                        n2599 = Wait (ms)(milliseconds to wait=u32 50) -> ()  [unwired: 1 out]
                      }
                      frame #21 {
                        n2600 = local read "Set Hz"() -> (w3826:dbl)
                        n2601 = Number To Fractional String(number=w3826, precision (6)=i16 2) -> (F-format string=w3825:string)  [unwired: 2 in]
                        n2602 = Concatenate Strings("Set Frequency [Hz] :" ("Content"), w3825) -> (w3828:string)
                        n2603 = local read "EVENT LOG"() -> (w3830:string)
                        n2604 = call "Event Log.vi"("Content"=w3828, "EVENT LOG"=w3830) -> ("EVENT LOG"=w3829:string)  [unwired: 8 in, 1 out]
                        n2605 = local write "EVENT LOG"(w3829) -> ()
                      }
                      frame #22 {
                        n2606 = Wait (ms)(milliseconds to wait=u32 50) -> ()  [unwired: 1 out]
                      }
                      frame #23 {
                        n2607 = local read "NORMAL LOAD"() -> (w3833:dbl)
                        n2608 = Number To Fractional String(number=w3833, precision (6)=i16 2) -> (F-format string=w3834:string)  [unwired: 2 in]
                        n2609 = Concatenate Strings("Applied Load [grams] :" ("Content"), w3834) -> (w3836:string)
                        n2610 = local read "EVENT LOG"() -> (w3838:string)
                        n2611 = call "Event Log.vi"("Content"=w3836, "EVENT LOG"=w3838) -> ("EVENT LOG"=w3837:string)  [unwired: 8 in, 1 out]
                        n2612 = local write "EVENT LOG"(w3837) -> ()
                      }
                      frame #24 {
                        n2613 = Wait (ms)(milliseconds to wait=u32 50) -> ()  [unwired: 1 out]
                      }
                      frame #25 {
                        n2614 = local read "Set Strk"() -> (w3841:dbl)
                        n2615 = Number To Fractional String(number=w3841, precision (6)=i16 2) -> (F-format string=w3842:string)  [unwired: 2 in]
                        n2616 = Concatenate Strings("Set Stroke [mm] :" ("Content"), w3842) -> (w3844:string)
                        n2617 = local read "EVENT LOG"() -> (w3846:string)
                        n2618 = call "Event Log.vi"("Content"=w3844, "EVENT LOG"=w3846) -> ("EVENT LOG"=w3845:string)  [unwired: 8 in, 1 out]
                        n2619 = local write "EVENT LOG"(w3845) -> ()
                      }
                      frame #26 {
                        n2620 = Wait (ms)(milliseconds to wait=u32 50) -> ()  [unwired: 1 out]
                      }
                      frame #27 {
                        n2621 = local read "Set Temp"() -> (w3849:dbl)
                        n2622 = Number To Fractional String(number=w3849, precision (6)=i16 2) -> (F-format string=w3850:string)  [unwired: 2 in]
                        n2623 = Concatenate Strings("Set Temperature [deg C] :" ("Content"), w3850) -> (w3852:string)
                        n2624 = local read "EVENT LOG"() -> (w3854:string)
                        n2625 = call "Event Log.vi"("Content"=w3852, "EVENT LOG"=w3854) -> ("EVENT LOG"=w3853:string)  [unwired: 8 in, 1 out]
                        n2626 = local write "EVENT LOG"(w3853) -> ()
                      }
                      frame #28 {
                        n2627 = Wait (ms)(milliseconds to wait=u32 50) -> ()  [unwired: 1 out]
                      }
                      frame #29 {
                        n2628 = local read "Set Rh"() -> (w3857:dbl)
                        n2629 = Number To Fractional String(number=w3857, precision (6)=i16 2) -> (F-format string=w3858:string)  [unwired: 2 in]
                        n2630 = Concatenate Strings("Set Humidity [%RH] :" ("Content"), w3858) -> (w3860:string)
                        n2631 = local read "EVENT LOG"() -> (w3862:string)
                        n2632 = call "Event Log.vi"("Content"=w3860, "EVENT LOG"=w3862) -> ("EVENT LOG"=w3861:string)  [unwired: 8 in, 1 out]
                        n2633 = local write "EVENT LOG"(w3861) -> ()
                      }
                      frame #30 {
                        n2634 = Wait (ms)(milliseconds to wait=u32 50) -> ()  [unwired: 1 out]
                      }
                      frame #31 {
                        n2635 = local read "test time"() -> (w3865:dbl)
                        n2636 = Number To Fractional String(number=w3865, precision (6)=i16 1) -> (F-format string=w3866:string)  [unwired: 2 in]
                        n2637 = Concatenate Strings("Test Duration [mins] :" ("Content"), w3866) -> (w3868:string)
                        n2638 = local read "EVENT LOG"() -> (w3870:string)
                        n2639 = call "Event Log.vi"("Content"=w3868, "EVENT LOG"=w3870) -> ("EVENT LOG"=w3869:string)  [unwired: 8 in, 1 out]
                        n2640 = local write "EVENT LOG"(w3869) -> ()
                      }
                      frame #32 {
                        w3871 = dbl[] [] ("History Data")
                        w3872 = cluster{"y":dbl, dbl, "y":dbl}[] [] ("History Data")
                        w3873 = FALSE ("Visible")
                        n2641 = property on="Stroke ( mm )" class="WFChart (strict)"("History Data"=w3872) -> ()  [unwired: 2 in, 2 out]
                        n2642 = property on="Humidity ( %RH )" class="WFChart (strict)"("History Data"=w3871) -> ()  [unwired: 2 in, 2 out]
                        n2643 = property on="Temperature ( Deg C )" class="WFChart (strict)"("History Data"=w3871) -> ()  [unwired: 2 in, 2 out]
                        n2644 = property on="Electrical Contact Resistance ( % )" class="WFChart (strict)"("History Data"=w3871) -> ()  [unwired: 2 in, 2 out]
                        n2645 = property on="Coefficient of Friction" class="WFChart (strict)"("History Data"=w3871) -> ()  [unwired: 2 in, 2 out]
                        n2646 = property on="Frictional Force ( N )" class="WFChart (strict)"("History Data"=w3871) -> ()  [unwired: 2 in, 2 out]
                        n2647 = property on="Coefficient of Friction" class="WFChart (strict)"("History Data"=w3871) -> ()  [unwired: 2 in, 2 out]
                        n2648 = property on="Frictional Force ( N )" class="WFChart (strict)"("History Data"=w3871) -> ()  [unwired: 2 in, 2 out]
                        n2649 = property on="Electrical Contact Resistance ( % )" class="WFChart (strict)"("History Data"=w3871) -> ()  [unwired: 2 in, 2 out]
                        n2650 = property on="Humidity ( %RH )" class="WFChart (strict)"("History Data"=w3871) -> ()  [unwired: 2 in, 2 out]
                        n2651 = property on="Stroke ( mm )" class="WFChart (strict)"("History Data"=w3872) -> ()  [unwired: 2 in, 2 out]
                        n2652 = property on="Temperature ( Deg C )" class="WFChart (strict)"("History Data"=w3871) -> ()  [unwired: 2 in, 2 out]
                        n2653 = property on="Service Password Log" class="Str"("Visible"=w3873) -> ()  [unwired: 2 in, 2 out]
                        n2654 = property on="Password 3" class="Clust (strict)"("Visible"=w3873) -> ()  [unwired: 2 in, 2 out]
                      }
                    }
                    "TEST FILE NAM,E SAVED" <- TRUE ("TEST FILE NAM,E SAVED")
